vi "get Name.vi"(11 "Timer in":refnum<class "Timer.lvclass">) -> (3 "Name":string)   [LabVIEW 2015, in "Timer.lvclass"]
uses:
  Timer.lvclass
  Timer.lvclass/Timer.ctl
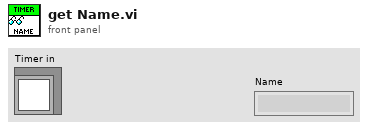
[diagram p1: front panel]
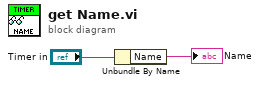
[diagram p0: block diagram]
diagram:
  n1 = Unbundle By Name("Timer in") -> ("Name"=→"Name":string)
